vi "IO_18v7Open.vi"() -> (0 "error out":errorcluster={"status"=TRUE, "code"=-1073807346, "source"="VISA Write in IO_18v7Open.vi"}, 3 "VISA Refnum out":refnum<visa-resource-name>)   [LabVIEW 2024]
uses:
  <vilib>/Instr/_visa.llb/VISA Configure Serial Port (Instr).vi
panel:
  out "ComPort Active":refnum<visa-resource-name>
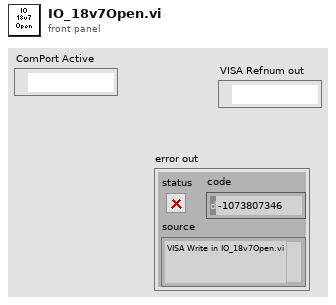
[diagram p1: front panel]
types:
  T1 = enum32{"invalid app kind", "Development System", "Run Time System", "Student Edition", "Embedded LabVIEW", "Evaluation", "Custom"}
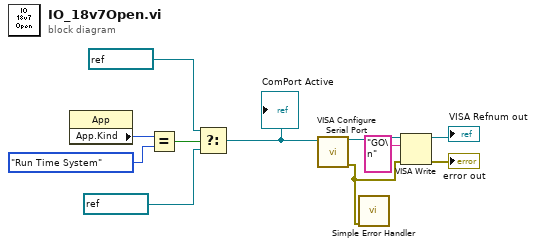
[diagram p0: block diagram]
diagram:
  n1 = property class="App"() -> ("App.Kind"=w6:T1)  [unwired: 2 in, 2 out]
  n2 = Equal?(x=w6, y=T1."Run Time System") -> (x = y?=w4:bool)
  n3 = Select(t=refnum<visa-resource-name> "COM5" ("VISA resource name"), s=w4, f=refnum<visa-resource-name> "COM4" ("VISA resource name")) -> (s? t:f=w1:refnum<visa-resource-name>)
  "ComPort Active" <- w1
  n4 = call-poly "VISA Configure Serial Port"("VISA resource name"=w1) -> ("VISA resource name out"=w7:refnum<visa-resource-name>, "error out"=w10:errorcluster)  [unwired: 13 in]
  n5 = call <vilib>:"Simple Error Handler.vi"("error in (no error)"=w10) -> ()  [unwired: 4 in, 5 out]
  n6 = VISA Write(VISA resource name=w7, write buffer="GO\n", error in (no error)=w10) -> (VISA resource name out=→"VISA Refnum out":refnum<visa-resource-name>, error out=→"error out":errorcluster)  [unwired: 1 out]
